vi "WFS Calc Wavefront Statistics.vi"(8 "error in (no error)":errorcluster {"code" format="%.0x"}, 11 "instrument handle":refnum<visa-resource-name>) -> (0 "error out":errorcluster {"code" format="%.0x"}, 1 "Max":dbl, 2 "Min":dbl, 3 "instrument handle out":refnum<visa-resource-name>, 4 "Diff":dbl, 5 "Mean":dbl, 6 "RMS":dbl, 7 "Weighted RMS":dbl)   [LabVIEW 2020]
doc: "This VI returns statistic parameters of the wavefront in µm calculated by WFS Calc Wavefront.vi.\n\nNote: WFS Calc Wavefront.vi is required to run prior to this VI."
uses:
  WFS_32.dll
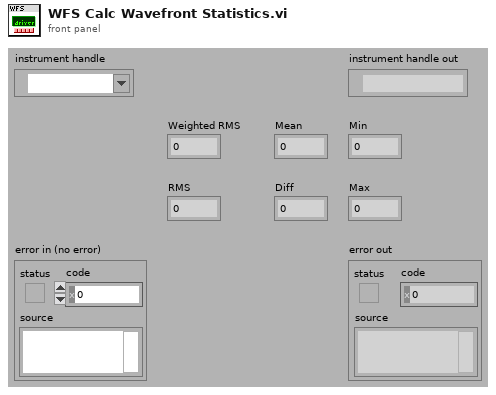
[diagram p1: front panel]
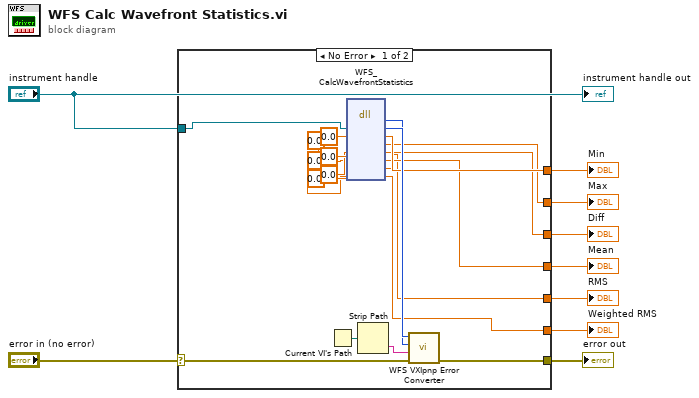
[diagram p0: block diagram]
diagram:
  n1 = case shown="No Error" "error in (no error)" {
    selector: "error in (no error)" -> [w23 w29]
    tunnel: [w22 w29] -> w9
    tunnel: "instrument handle" -> [w27 _]
    tunnel: [w20 _] -> w6
    tunnel: [w18 _] -> w5
    tunnel: [w16 _] -> w4
    tunnel: [w14 _] -> w3
    tunnel: [w12 _] -> w2
    tunnel: [w10 _] -> w1
    frame No Error {
      n2 = Current VI's Path() -> (path=w28:path)
      n3 = dll-call lib="WFS_*.*" fn="WFS_CalcWavefrontStatistics"("Instrument Handle"=w27, "Min"=0.0, "Max"=0.0, "Diff"=0.0, "Mean"=0.0, "RMS"=0.0, "Weighted RMS"=0.0) -> (w25:i32, "Instrument Handle"=w26:u32, "Min"=w20:dbl, "Max"=w18:dbl, "Diff"=w16:dbl, "Mean"=w14:dbl, "RMS"=w12:dbl, "Weighted RMS"=w10:dbl)  [unwired: 3 in, 2 out]
      n4 = Strip Path(path=w28) -> (name=w24:string)  [unwired: 1 out]
      n5 = call "WFS VXIpnp Error Converter.vi"("error in (no error)"=w23, "Name Of VI (\"\")"=w24, "CVI Error Code (0)"=w25, "instrument handle"=w26) -> ("error out"=w22:errorcluster)  [unwired: 6 in, 1 out]
    }
    frame Error {
    }
  }
  "error out" <- w9
  "Min" <- w6
  "Max" <- w5
  "Diff" <- w4
  "Mean" <- w3
  "RMS" <- w2
  "Weighted RMS" <- w1
  "instrument handle out" <- "instrument handle"
